vi "Relay Actor Broadcast Msg.vi"(8 "error in (no error)":errorcluster, 10 "Caller Enqueuer":refnum<class "Message Enqueuer.lvclass">, 11 "ActorEventMessage In":refnum<class "Abstract Broadcast Data Msg.lvclass">) -> (0 "error out":errorcluster)   [LabVIEW 2015, in "IViewable.lvlib" / "Abstract Broadcast Data Msg.lvclass"]
uses:
  Abstract Broadcast Data Msg.lvclass
  <vilib>/ActorFramework/Message Enqueuer/Message Enqueuer.lvclass
  <vilib>/ActorFramework/Message Enqueuer/Message Enqueuer.lvclass/Message Enqueuer.ctl
  <vilib>/ActorFramework/Message Priority Queue/Priority Enqueue.vi
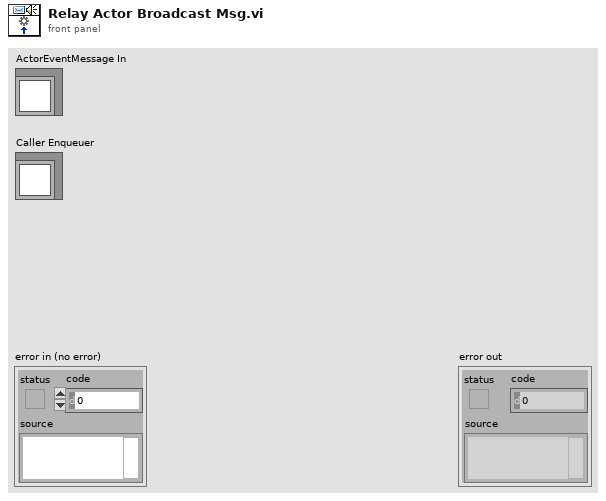
[diagram p1: front panel]
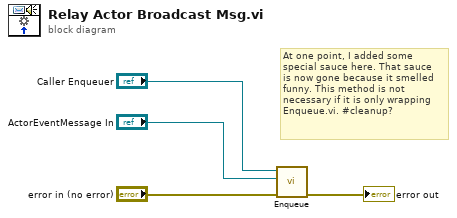
[diagram p0: block diagram]
diagram:
  # "At one point, I added some\nspecial sauce here. That sauce\nis now gone because it smelled\nfunny. This method is not\nnecessary if it is only wrapping\nEnqueue.vi. #cleanup?"
  n1 = call <vilib>:"Enqueue.vi"("error in (no error)"="error in (no error)", "Message"="ActorEventMessage In", "Message Enqueuer in"="Caller Enqueuer") -> ("error out"=→"error out":errorcluster)  [unwired: 7 in, 1 out]
